vi "Create_Object.vi"(8 "error in (no error)":errorcluster, 9 "Terminal Map in":map{string, T1}(c390), 10 "owner refnum":variant, 11 "Bool Control in":refnum<class "Bool Control.lvclass">) -> (0 "error out":errorcluster, 1 "Terminal Map Out":map{string, T1}(c390), 3 "Bool Control out":refnum<class "Bool Control.lvclass">)   [LabVIEW 2025, in "Bool Control.lvclass"]
uses:
  Bool Control.lvclass
  Controls/Terminal.ctl
  Node.lvclass/Node.ctl
  Control.lvclass
  Node.lvclass
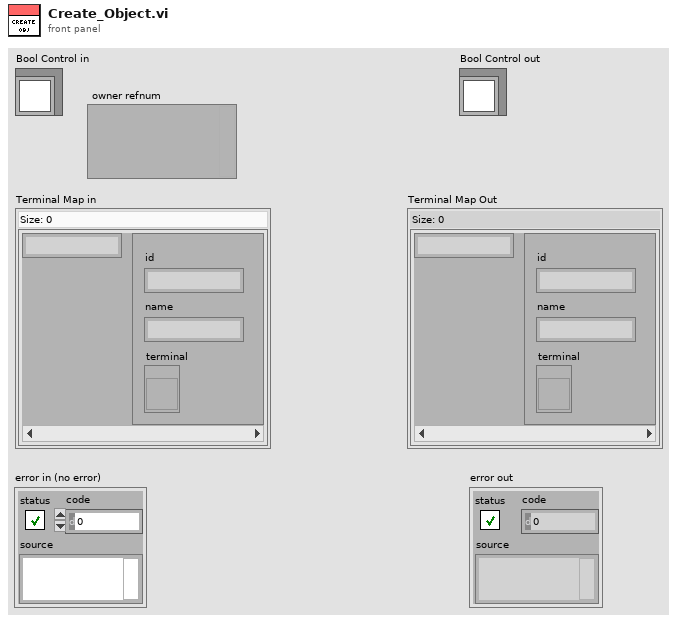
[diagram p1: front panel]
types:
  T1 = typedef "Terminal.ctl" = cluster{"id":string, "name":string, "terminal":refnum<vi>}
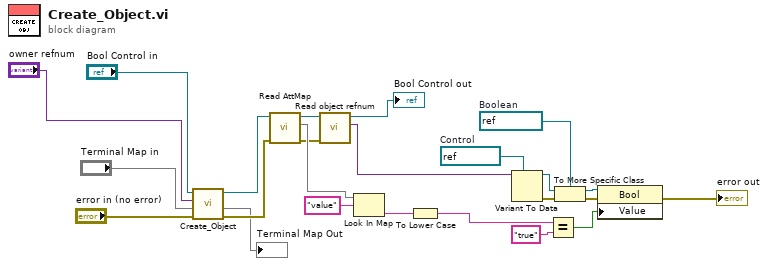
[diagram p0: block diagram]
diagram:
  w19 = refnum<vi> refnum  # Boolean
  w20 = refnum<vi> refnum  # Control
  n1 = call-parent "Create_Object.vi"("error in (no error)"="error in (no error)", "Terminal Map in"="Terminal Map in", "owner refnum"="owner refnum", "Control in"="Bool Control in") -> ("error out"=w10:errorcluster, "Terminal Map Out"=→"Terminal Map Out":map{string, T1}, "Control out"=w11:refnum<class "Bool Control.lvclass">)  [unwired: 5 in]
  n2 = call "Read AttMap.vi"("error in (no error)"=w10, "Node in"=w11) -> ("error out"=w8:errorcluster, "AttMap"=w9:map{string, string}, "Node out"=w7:refnum<class "Bool Control.lvclass">)  [unwired: 7 in]
  n3 = call-dynamic "Read object refnum.vi"("error in (no error)"=w8, "Node in"=w7) -> ("object refnum"=w6:variant, "Node out"=→"Bool Control out":refnum<class "Bool Control.lvclass">)  [unwired: 7 in, 1 out]
  n4 = Look In Map(map=w9, key="value" ("valueConst")) -> (value=w14:string)  [unwired: 1 in, 1 out]
  n5 = To Lower Case(string=w14) -> (all lower case string=w1:string)
  n6 = Variant To Data(type=w20, Variant=w6) -> (data=w18:refnum<vi>, error out=w17:errorcluster)  [unwired: 1 in]
  n7 = Equal?(x=w1, y="true" ("compareConst")) -> (x = y?=w12:bool)
  n8 = To More Specific Class(target class=w19, reference=w18, error in=w17) -> (specific class reference=w21:refnum<vi>, error out=w16:errorcluster)
  n9 = property class="Bool"(reference=w21, error in=w16, "Value"=w12) -> (error out=→"error out":errorcluster)  [unwired: 1 out]
